vi "TDMS.GetChannelsForLevelTransitionAnalysis.vi"(8 "error in (no error)":errorcluster, 11 "TDMS Ref":refnum<k34>) -> (0 "error out":errorcluster, 1 "ODH Channels":string[](array[string]), 2 "OPH Channels":string[](array[string]), 3 "TDMS Ref out":refnum<k34>)   [LabVIEW 2014, in "NIAnalysis.lvlib"]
uses:
  NIAnalysis.lvlib
  Constants.vi
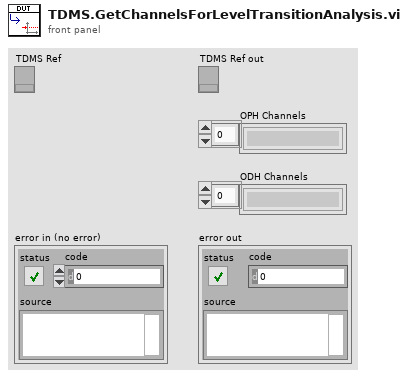
[diagram p1: front panel]
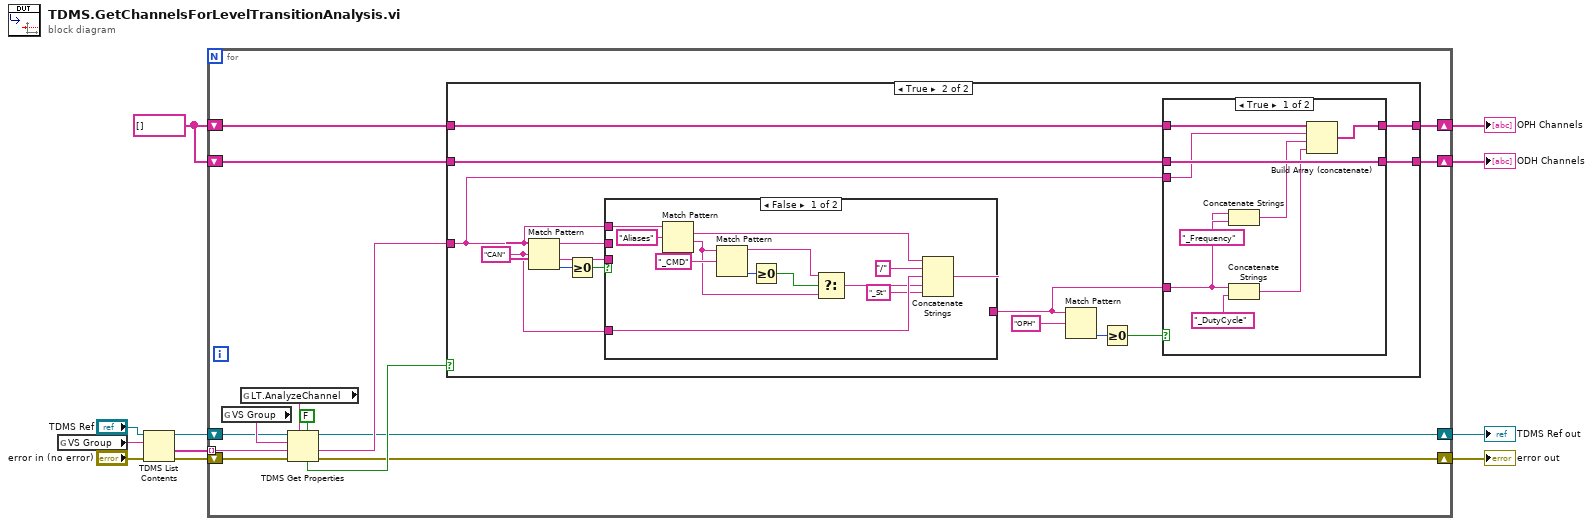
[diagram p0: block diagram]
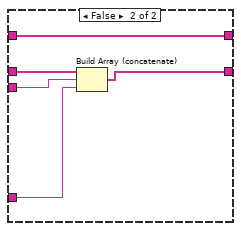
[diagram p3: hidden frame]
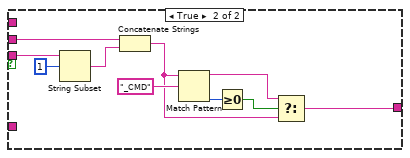
[diagram p4: hidden frame]
diagram:
  w7 = string[] []
  n1 = global read "Constants.vi" "VS Group"() -> (w6:string)
  n2 = TDMS List Contents(4:"error in (no error)", 6:w6, 7:"TDMS Ref") -> (0:w1:errorcluster, 1:w5:string[], 3:w3:refnum<k34>)  [unwired: 1 out]
  n3 = for {
    shift-right: [w22] -> w9
    shift-left: w7 -> [w25]
    shift-right: [w23] -> w8
    shift-left: w7 -> [w24]
    tunnel: w5 -> [w19] mode=indexing
    shift-right: [w14] -> w10
    shift-left: w3 -> [w15]
    shift-right: [w12] -> w11
    shift-left: w1 -> [w13]
    n4 = global read "Constants.vi" "VS Group"() -> (w18:string)
    n5 = global read "Constants.vi" "LT.AnalyzeChannel"() -> (w21:string)
    n6 = TDMS Get Properties(5:FALSE, 7:w21, 8:w13, 9:w19, 10:w18, 11:w15) -> (0:w12:errorcluster, 1:w16:string, 3:w14:refnum<k34>, 4:w17:bool)  [unwired: 2 out]
    n7 = case shown="True" w17 {
      tunnel: w16 -> [_ w28]
      tunnel: w25 -> [w27 w32]
      tunnel: w24 -> [w26 w31]
      tunnel: [w26 w30] -> w23
      tunnel: [w27 w29] -> w22
      frame False {
      }
      frame True {
        w37 = "CAN" ("regular expression")
        n8 = Match Pattern(string=w28, regular expression=w37) -> (before substring=w39:string, after substring=w38:string, offset past match=w41:i32)  [unwired: 1 in, 1 out]
        n9 = Greater Or Equal To 0?(x=w41) -> (x >= 0?=w40:bool)
        n10 = case shown="False" w40 {
          tunnel: w39 -> [_ w75]
          tunnel: w38 -> [_ w77]
          tunnel: [w63 w69] -> w34
          tunnel: w28 -> [w68 _]
          tunnel: w37 -> [w66 _]
          frame False {
            n11 = Match Pattern(string=w68, regular expression="Aliases") -> (match substring=w64:string, after substring=w57:string)  [unwired: 1 in, 2 out]
            n12 = Match Pattern(string=w57, regular expression="_CMD") -> (before substring=w58:string, offset past match=w60:i32)  [unwired: 1 in, 2 out]
            n13 = Greater Or Equal To 0?(x=w60) -> (x >= 0?=w59:bool)
            n14 = Select(t=w58, s=w59, f=w57) -> (s? t:f=w56:string)
            n15 = Concatenate Strings(w64, "/" ("string"), w66, w56, "_St" ("string")) -> (w63:string)
          }
          frame True {
            n16 = String Subset(string=w77, offset (0)=1) -> (substring=w76:string)  [unwired: 1 in]
            n17 = Concatenate Strings(w75, w76) -> (w70:string)
            n18 = Match Pattern(string=w70, regular expression="_CMD") -> (before substring=w71:string, offset past match=w73:i32)  [unwired: 1 in, 2 out]
            n19 = Greater Or Equal To 0?(x=w73) -> (x >= 0?=w72:bool)
            n20 = Select(t=w71, s=w72, f=w70) -> (s? t:f=w69:string)
          }
        }
        n21 = Match Pattern(string=w34, regular expression="OPH") -> (offset past match=w35:i32)  [unwired: 1 in, 3 out]
        n22 = Greater Or Equal To 0?(x=w35) -> (x >= 0?=w33:bool)
        n23 = case shown="True" w33 {
          tunnel: w34 -> [w48 w54]
          tunnel: w28 -> [w45 w55]
          tunnel: w32 -> [w46 w51]
          tunnel: w31 -> [w47 w53]
          tunnel: [w47 w52] -> w30
          tunnel: [w42 w51] -> w29
          frame True {
            n24 = Concatenate Strings(w48, "_Frequency" ("string")) -> (w44:string)
            n25 = Concatenate Strings(w48, "_DutyCycle" ("string")) -> (w43:string)
            n26 = Build Array (concatenate)(w46, w45, w44, w43) -> (w42:string[])
          }
          frame False {
            n27 = Build Array (concatenate)(w53, w55, w54) -> (w52:string[])
          }
        }
      }
    }
  }
  "error out" <- w11
  "TDMS Ref out" <- w10
  "OPH Channels" <- w9
  "ODH Channels" <- w8
